vi "Demo_Modbus.vi"() -> ()   [LabVIEW 2016]
uses:
  <vilib>/Modbus/master/Modbus Master.lvclass
  CommandAndControl-main/Experiment_pump_for FR_Updated/database/database.lvlib
  <vilib>/Modbus/master/Create Master Instance (Serial).vi
panel:
  out "JSON字符串":string
  in  "启动时间（毫秒）":u32
  in  "dataLabel":string
  in  "msg_id":dbl
  out "当前指令":string
  out "json error":errorcluster caption="JSON Error"
  out "波形图表 2":dynamicdata(graph)
  in  "JSON parser":T1
  in  "参考电阻_ITO":dbl
  in  "总压降":dbl=65535.0
  in  "参考电阻":dbl[](array[numeric])
  in  "TestId":string
  out "coil values":bool[](array[boolean]) caption="线圈值"
  out "AIn":u16[](array[numeric]) caption="寄存器值"
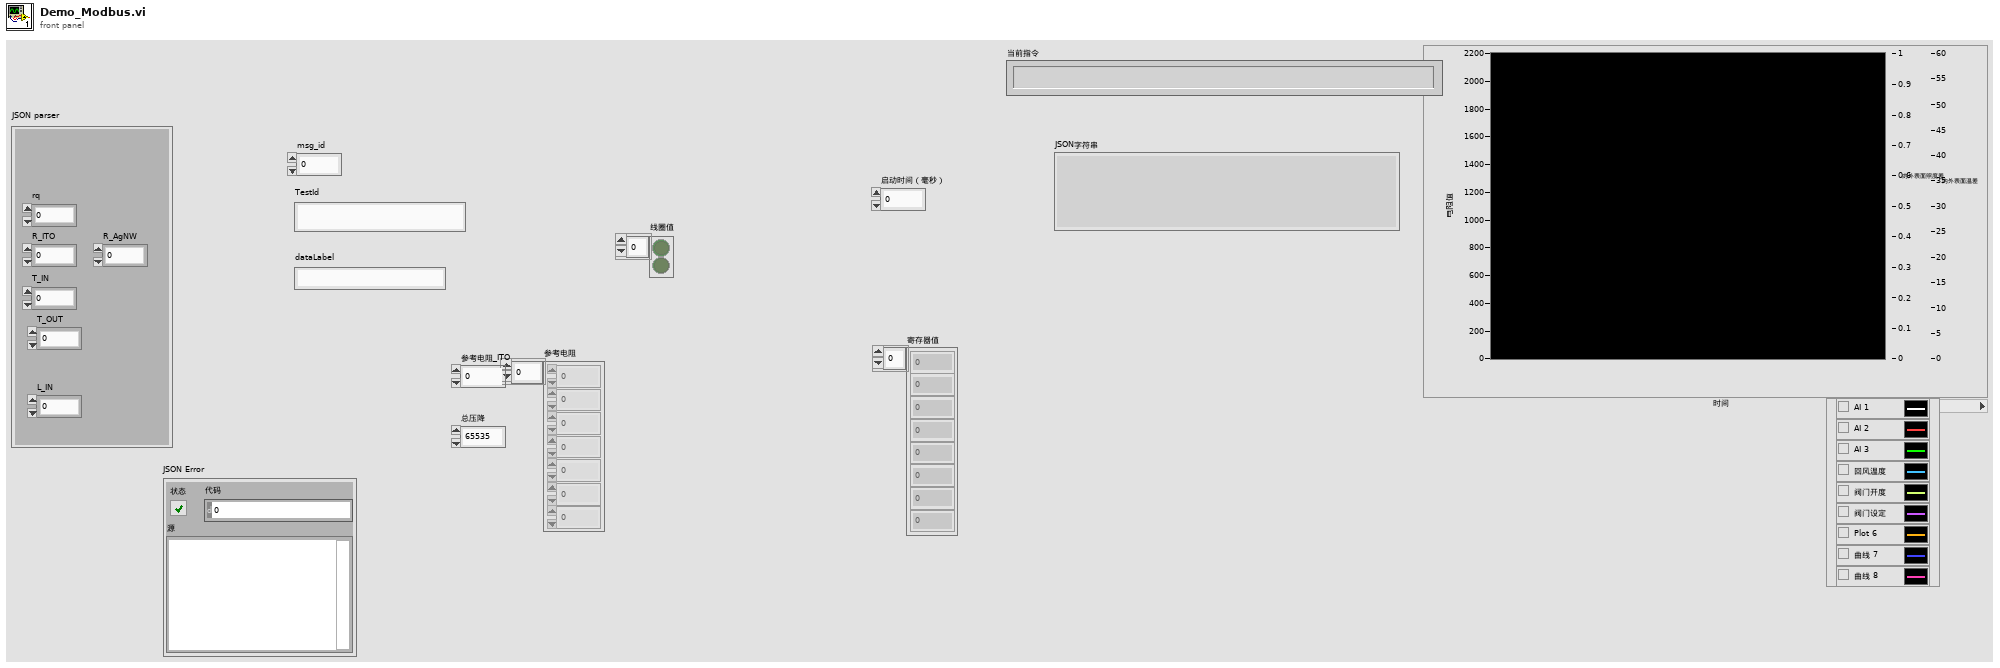
[diagram p1: front panel]
types:
  T1 = cluster{"rq":dbl, "R_ITO":dbl, "T_IN":dbl, "T_OUT":dbl, "R_AgNW":dbl, "L_IN":dbl}
  T2 = cluster{"NewVal[0]":u16, "NewVal[1]":u16, "NewVal[2]":u16, "NewVal[3]":u16, "NewVal[4]":u16, "NewVal[5]":u16, "NewVal[6]":u16, "NewVal[7]":u16, "NewVal[8]":u16}
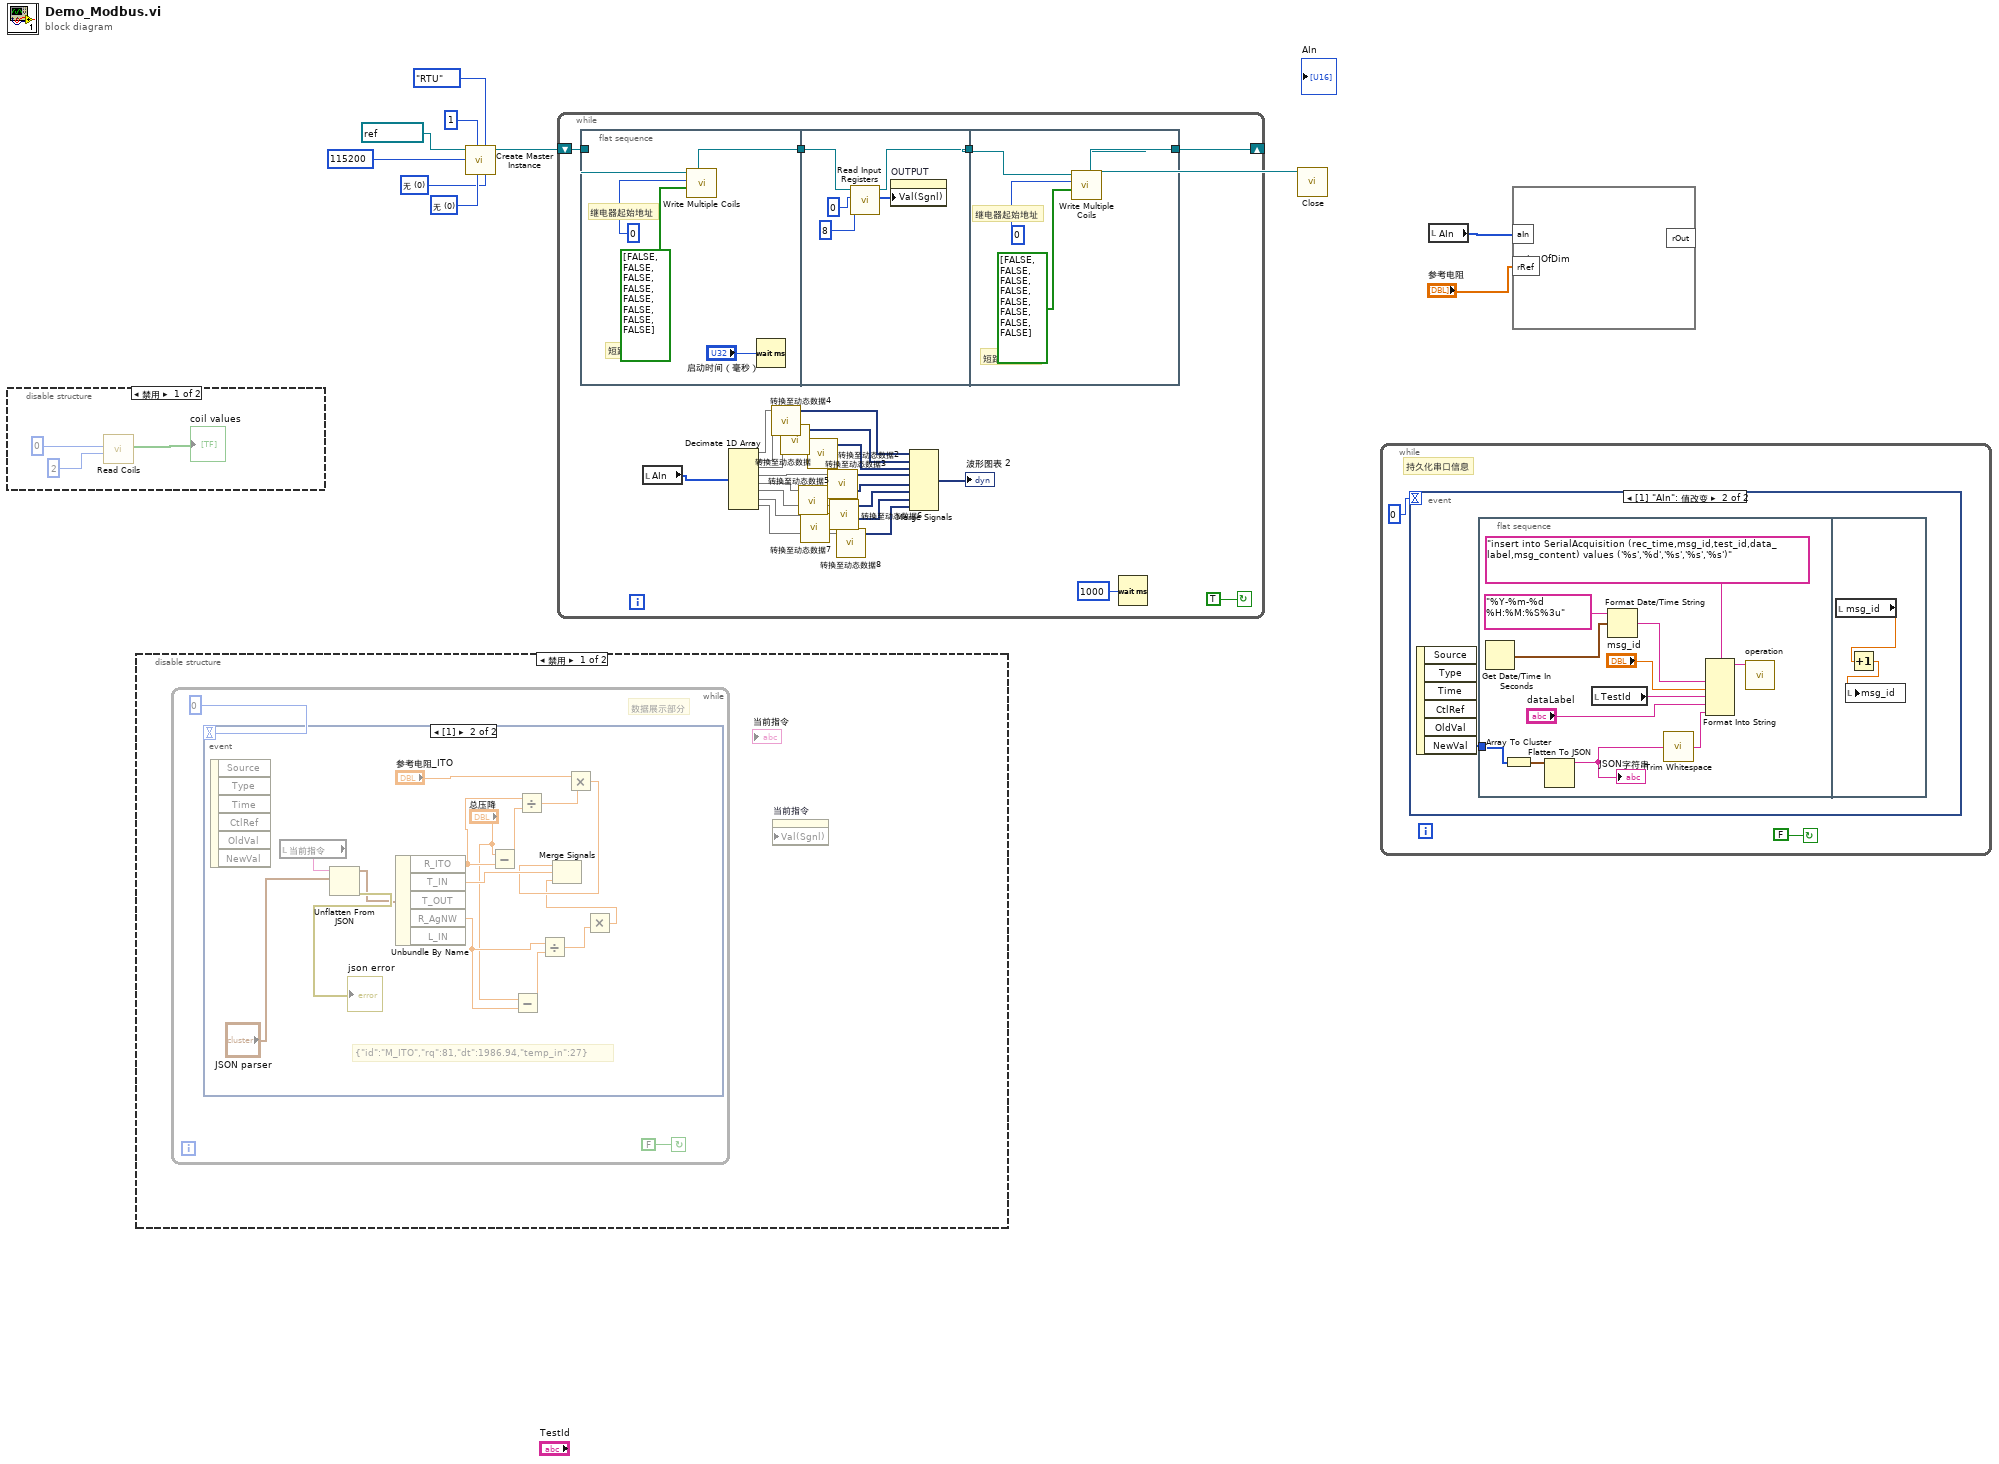
[diagram p0: block diagram]
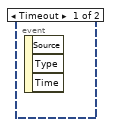
[diagram p2: hidden frame]
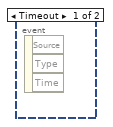
[diagram p3: hidden frame]
diagram:
  w5 = u16 0 items=["无", "XON/XOFF", "RTS/CTS", "XON/XOFF & RTS/CTS", "DTR/DSR", "XON/XOFF & DTR/DSR"] ("flow control (None)")
  w6 = u16 0 items=["无", "奇", "偶"] ("parity (Even)")
  n1 = disable-structure shown="禁用" {
    frame Disabled {
      n2 = call-dynamic "Read Coils.vi"("number of coils"=u16 2, "starting address"=u16 0) -> ("coil values"=→"coil values":bool[], "Modbus master out"=w13:refnum<class "Modbus Master.lvclass">)  [unwired: 7 in, 1 out]
    }
    frame Enabled {
    }
  }
  n3 = disable-structure shown="禁用" {
    frame Disabled {
      n4 = while {
        stop <- FALSE continue-if-true
        # "数据展示部分"
        n5 = event shown="[1]" {
          selector: _ -> [_ _]
          dyn-events: _ -> [_ _]
          timeout: 0 -> [_ _]
          event Timeout {
            n6 = event-data() -> ()  [unwired: 1 in, 3 out]
          }
          event #1 (no event record) {
            # "{\"id\":\"M_ITO\",\"rq\":81,\"dt\":1986.94,\"temp_in\":27}"
            n7 = event-data() -> ()  [unwired: 1 in, 6 out]
            n8 = local read "当前指令"() -> (w31:string)
            n9 = Unflatten From JSON(JSON string=w31, type and defaults="JSON parser") -> (value=w29:T1, error out=→"json error":errorcluster)  [unwired: 5 in]
            n10 = Unbundle By Name(w29) -> ("R_ITO"=w26:dbl, "T_IN"=w28:dbl, "R_AgNW"=w19:dbl)  [unwired: 2 out]
            n11 = Subtract(x="总压降", y=w26) -> (x-y=w25:dbl)
            n12 = Subtract(x="总压降", y=w19) -> (x-y=w21:dbl)
            n13 = Divide(x=w26, y=w25) -> (x/y=w24:dbl)
            n14 = Divide(x=w19, y=w21) -> (x/y=w20:dbl)
            n15 = Multiply(x="参考电阻_ITO", y=w24) -> (x*y=w22:dbl)
            n16 = Multiply(y=w20) -> (x*y=w17:dbl)  [unwired: 1 in]
            n17 = Merge Signals(w22, w28, w17) -> ()  [unwired: 1 out]
          }
        }
      }
      n18 = property on="当前指令" class="Str" props=["Val(Sgnl)"]() -> ()  [unwired: 3 in, 2 out]
    }
    frame Enabled {
    }
  }
  n19 = call-poly <vilib>:"Create Master Instance.vi"("flow control (None)"=w5, "serial type"=enum16{"RTU", "ASCII"}."RTU", "parity (Even)"=w6, "unit ID"=u8 1, "baud rate (9600)"=u32 115200, "VISA resource name"=refnum<visa-resource-name> "COM5") -> ("serial master instance"=w4:refnum<class "Modbus Master.lvclass">)  [unwired: 4 in, 1 out]
  n20 = while {
    shift-right: [w54] -> w3
    shift-left: w4 -> [w55]
    stop <- TRUE continue-if-true
    n21 = flat-sequence {
      tunnel: w55 -> [w60]
      tunnel: [w59] -> w52
      tunnel: w52 -> [w63]
      tunnel: [w62] -> w51
      tunnel: [w66] -> w54
      tunnel: w51 -> [w67]
      frame #0 {
        # "短路口全断开"
        # "继电器起始地址"
        n22 = call-dynamic "Write Multiple Coils.vi"("coil values"=bool[] [FALSE, FALSE, FALSE, FALSE, FALSE, FALSE, FALSE, FALSE], "starting address"=u16 0, "Modbus master in"=w60) -> ("Modbus master out"=w59:refnum<class "Modbus Master.lvclass">)  [unwired: 7 in, 1 out]
        n23 = Wait (ms)(milliseconds to wait="启动时间（毫秒）") -> ()  [unwired: 1 out]
      }
      frame #1 {
        n24 = call-dynamic "Read Input Registers.vi"("number of input registers"=u16 8 ("number of holding registers"), "starting address"=u16 0, "Modbus master in"=w63) -> ("register values"=w61:u16[], "Modbus master out"=w62:refnum<class "Modbus Master.lvclass">)  [unwired: 6 in, 1 out]
        n25 = property on="OUTPUT" class="Arr (严格)"("Val(Sgnl)"=w61) -> ()  [unwired: 2 in, 2 out]
      }
      frame #2 {
        # "短路线全闭合"
        # "继电器起始地址"
        n26 = call-dynamic "Write Multiple Coils.vi"("coil values"=bool[] [FALSE, FALSE, FALSE, FALSE, FALSE, FALSE, FALSE, FALSE], "starting address"=u16 0, "Modbus master in"=w67) -> ("Modbus master out"=w66:refnum<class "Modbus Master.lvclass">)  [unwired: 7 in, 1 out]
      }
    }
    n27 = local read "AIn"() -> (w32:u16[])
    n28 = Decimate 1D Array(w32) -> (w33:u16[], w35:u16[], w37:u16[], w39:u16[], w41:u16[], w43:u16[], w45:u16[], w47:u16[])
    n29 = call "转换至动态数据4"("Array"=w33) -> ("Dynamic Data Type"=w34:dynamicdata)  [unwired: 3 in]
    n30 = call "转换至动态数据"("Array"=w35) -> ("Dynamic Data Type"=w36:dynamicdata)  [unwired: 3 in]
    n31 = call "转换至动态数据5"("Array"=w41) -> ("Dynamic Data Type"=w42:dynamicdata)  [unwired: 3 in]
    n32 = call "转换至动态数据7"("Array"=w45) -> ("Dynamic Data Type"=w46:dynamicdata)  [unwired: 3 in]
    n33 = call "转换至动态数据2"("Array"=w37) -> ("Dynamic Data Type"=w38:dynamicdata)  [unwired: 3 in]
    n34 = call "转换至动态数据3"("Array"=w39) -> ("Dynamic Data Type"=w40:dynamicdata)  [unwired: 3 in]
    n35 = call "转换至动态数据6"("Array"=w43) -> ("Dynamic Data Type"=w44:dynamicdata)  [unwired: 3 in]
    n36 = call "转换至动态数据8"("Array"=w47) -> ("Dynamic Data Type"=w48:dynamicdata)  [unwired: 3 in]
    n37 = Merge Signals(w34, w36, w38, w40, w42, w44, w46, w48) -> (→"波形图表 2":dynamicdata)
    n38 = Wait (ms)(milliseconds to wait=u32 1000 ("等待时间（毫秒）")) -> ()  [unwired: 1 out]
  }
  n39 = call-dynamic "Close.vi"("Modbus master in"=w3) -> ()  [unwired: 10 in, 1 out]
  n40 = while {
    stop <- FALSE continue-if-true
    # "持久化串口信息"
    n41 = event shown="[1] \"AIn\": 值改变" {
      selector: _ -> [_ _]
      dyn-events: _ -> [_ _]
      timeout: 0 -> [_ _]
      event Timeout {
        n42 = event-data() -> ()  [unwired: 1 in, 3 out]
      }
      event "AIn": Value Change {
        n43 = event-data() -> ("NewVal"=w72:u16[])  [unwired: 1 in, 5 out]
        n44 = flat-sequence {
          tunnel: w72 -> [w73]
          frame #0 {
            n45 = Get Date/Time In Seconds() -> (seconds since 1Jan1904=w82:timestamp)
            n46 = Array To Cluster(array=w73) -> (cluster=w75:T2)
            n47 = Flatten To JSON(anything=w75) -> (JSON string=w74:string)  [unwired: 2 in, 1 out]
            "JSON字符串" <- w74
            n48 = local read "TestId"() -> (w78:string)
            n49 = Format Date/Time String ("格式化日期/时间字符串")(time format string (%c)="%Y-%m-%d %H:%M:%S%3u" ("时间格式字符串(%c)"), seconds (now)=w82) -> (date/time string=w79:string)  [unwired: 1 in]
            n50 = call <vilib>:"Trim Whitespace.vi"("string"=w74) -> ("trimmed string"=w80:string)  [unwired: 1 in]
            n51 = Format Into String(format string="insert into SerialAcquisition (rec_time,msg_id,test_id,data_label,msg_content) values ('%s','%d','%s','%s','%s')" ("格式字符串"), w79, "msg_id", w78, "dataLabel", w80) -> (resulting string=w81:string)  [unwired: 2 in, 1 out]
            n52 = call "operation.vi"("Command Text"=w81) -> ()  [unwired: 9 in, 1 out]
          }
          frame #1 {
            n53 = local read "msg_id"() -> (w86:dbl)
            n54 = Increment(x=w86) -> (x+1=w85:dbl)
            n55 = local write "msg_id"(w85) -> ()
          }
        }
      }
    }
  }
  n56 = local read "AIn"() -> (w2:u16[])
  n57 = formula code="sizeOfDim"("aIn"=w2, "rRef"="参考电阻") -> ()  [unwired: 1 out]
